vi "SV UFF58 Write ASCII Function.vi"   [LabVIEW 2017, in "SoundVib_UFF58.lvlib"]
doc: "Writes data to the UFF58 (universal file format) file specified by the <B>file refnum</B> input. This VI also writes the fields in records 1, 2, and 3, <B>ID lines (1-3)</B>. You can write a single time domain waveform, a single real frequency spectrum, or a complex frequency spectrum to a UFF file. If a frequency spectrum is in decibels, this VI converts the spectrum to linear before writing to the UFF58 file. The default instance, SV UFF58 Write ASCII Function (Time Waveform), writes a single time domain waveform to the file specified by the <B>file refnum</B> input. Wire data to the <B>file refnum</B> input to determine the polymorphic instance to use or manually select the instance."
uses:
  <vilib>/addons/Sound and Vibration/svt_UFF58/SoundVib_UFF58.lvlib
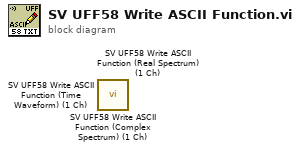
[diagram p0: block diagram]
diagram:
  n1 = call <vilib>:"SV UFF58 Write ASCII Function (Complex Spectrum) (1 Ch).vi"() -> ()  [unwired: 14 in, 2 out]
  n2 = call <vilib>:"SV UFF58 Write ASCII Function (Real Spectrum) (1 Ch).vi"() -> ()  [unwired: 14 in, 2 out]
  n3 = call <vilib>:"SV UFF58 Write ASCII Function (Time Waveform) (1 Ch).vi"() -> ()  [unwired: 14 in, 2 out]
